vi "scale U8 values for colour.vi"(8 "error in (no error)":errorcluster, 11 "U8 Values":u8[](array[numeric])) -> (0 "error out":errorcluster, 3 "scaled U8":sgl[](array[numeric]))   [LabVIEW 2020]
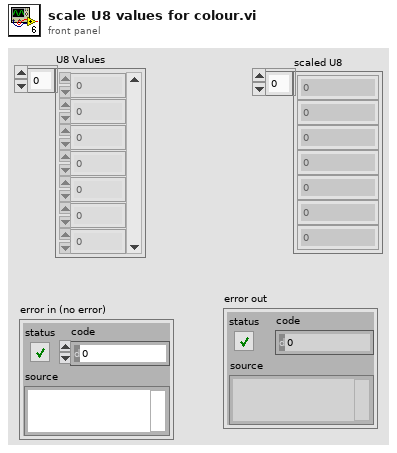
[diagram p1: front panel]
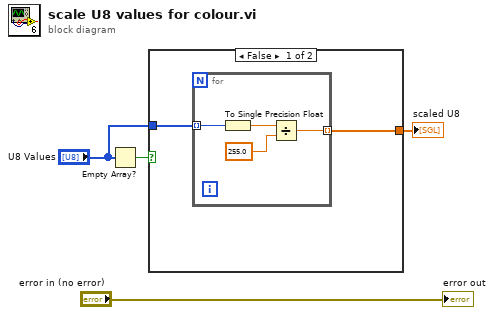
[diagram p0: block diagram]
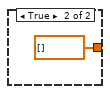
[diagram p2: hidden frame]
diagram:
  n1 = Empty Array?(array="U8 Values") -> (empty?=w4:bool)
  n2 = case shown="False" w4 {
    tunnel: "U8 Values" -> [w6 _]
    tunnel: [w5 sgl[] []] -> w2
    frame False {
      n3 = for {
        tunnel: w6 -> [w10] mode=indexing
        tunnel: [w7] -> w5 mode=indexing
        n4 = To Single Precision Float(number=w10) -> (single precision float=w9:sgl)
        n5 = Divide(x=w9, y=sgl 255.0) -> (x/y=w7:sgl)
      }
    }
    frame True {
    }
  }
  "scaled U8" <- w2
  "error out" <- "error in (no error)"
